vi "Datalog V1.0.vi"(11 "notifiers in":T1) -> ()   [LabVIEW 2022 SP3]
uses:
  Controls/All Notifer.ctl
  Controls/UI Data.ctl
  Controls/Datalog Control.ctl
  Controls/Root path.ctl
  Controls/All Loop Status.ctl
  Sub VI's/Global 1.vi
panel:
  out "error in":errorcluster
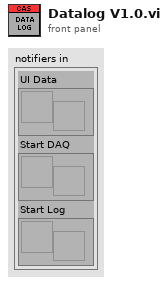
[diagram p1: front panel]
types:
  T1 = typedef "All Notifer.ctl" = cluster{"UI Data":refnum<notifier>, "Start DAQ":refnum<notifier>, "Start Log":refnum<notifier>}
  T2 = typedef "Root path.ctl" = cluster{"Data":path, "Sub VI's":path, "Source code":path}
  T3 = cluster{"in progress?":bool, "DI_ref":refnum<queue>, "Start Log":refnum<notifier>, "tdms ref":refnum<k34>, "AI\nAO\nDO\nTC\nACC\nStrain":refnum<queue>[], "Root Path":T2, "Start time":timestamp}
  T4 = typedef "Datalog Control.ctl" = enum16{"Init", "Poll", "Flush Qs", "Create File", "Log AI", "Log DI", "Log DO", "Log AO", "Close File", "Error", "Exit"}
  T5 = typedef "All Loop Status.ctl" = enum16{"AI", "AO", "DI", "DO", "TC", "Strain", "ACC", "RT", "Log", "Seq", "Sync"}
  T6 = enum16{"Init", "Read 'All'", "Read 'n'", "Read '1'", "Write '1'", "Write 'n'", "Write 'All'"}
  T7 = enum16{"open", "open or create", "create or replace", "create", "open (read-only)"}
  T8 = typedef "All Queue.ctl" = cluster{"AI\nAO\nDO\nTC\nACC\nStrain":refnum<queue>[], "DI":refnum<queue>}
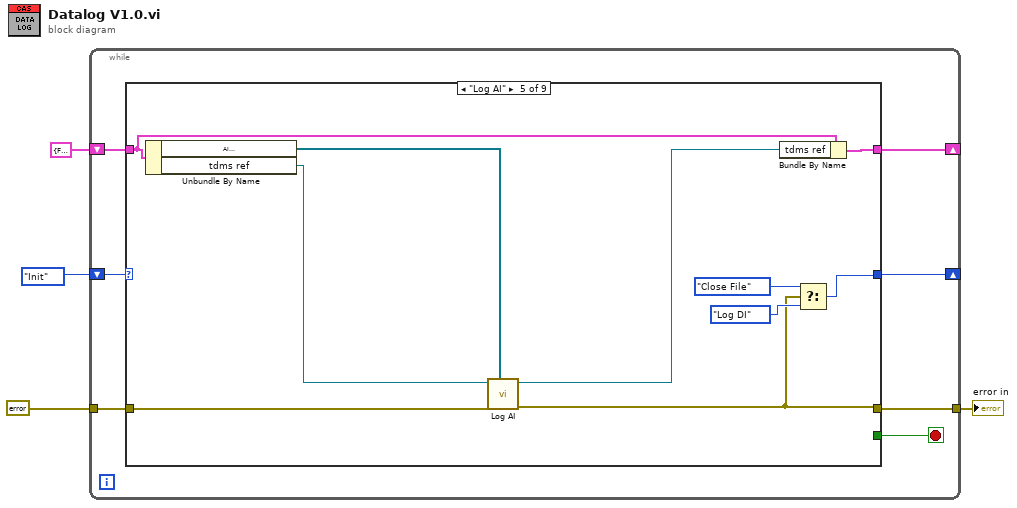
[diagram p0: block diagram]
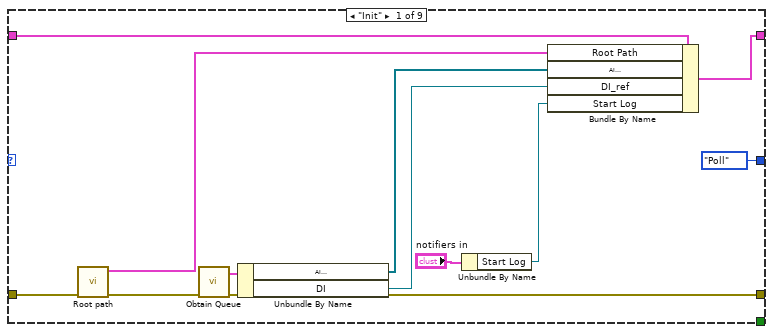
[diagram p2: hidden frame]
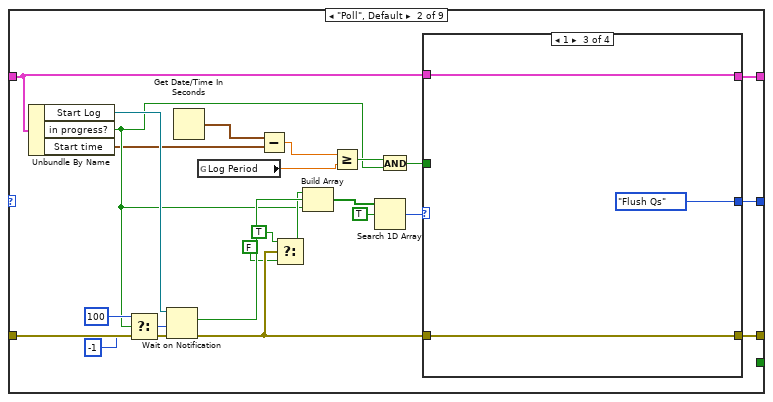
[diagram p3: hidden frame]
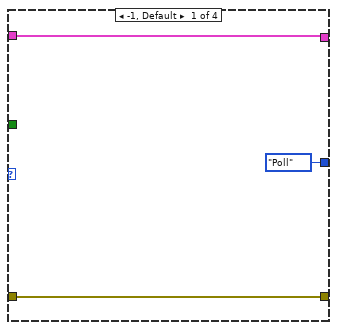
[diagram p4: hidden frame]
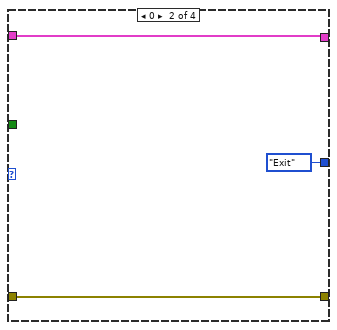
[diagram p5: hidden frame]
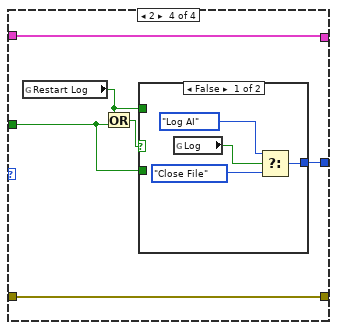
[diagram p6: hidden frame]
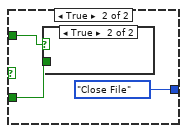
[diagram p7: hidden frame]
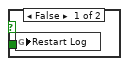
[diagram p8: hidden frame]
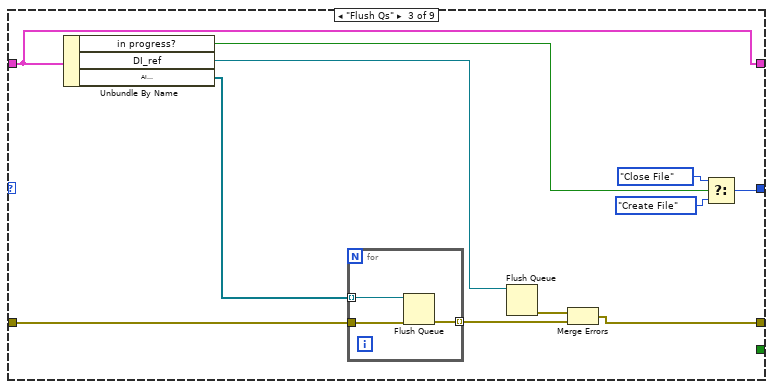
[diagram p9: hidden frame]
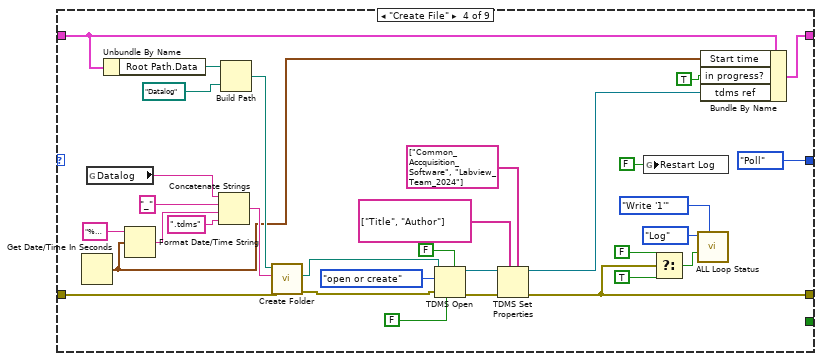
[diagram p10: hidden frame]
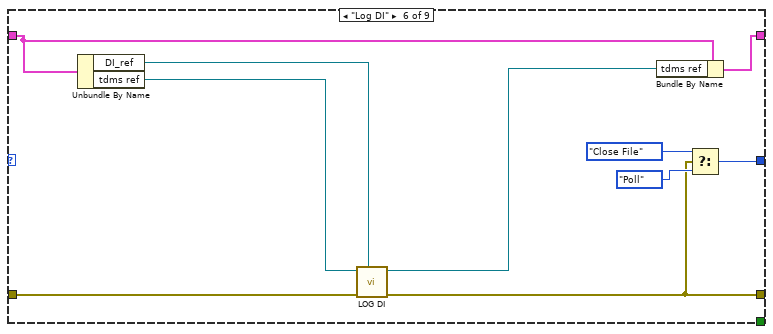
[diagram p11: hidden frame]
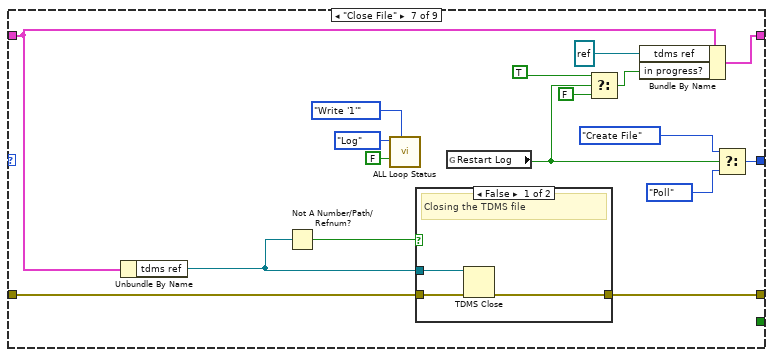
[diagram p12: hidden frame]
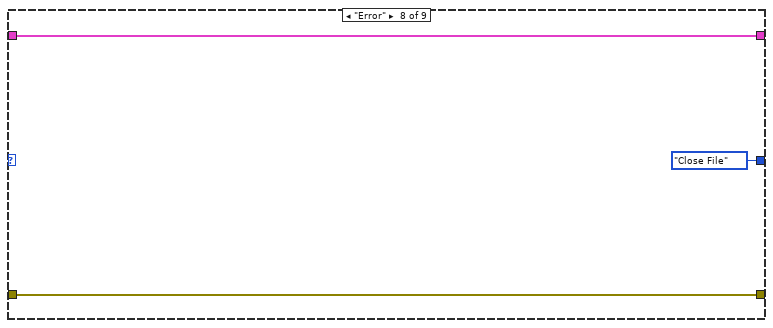
[diagram p14: hidden frame]
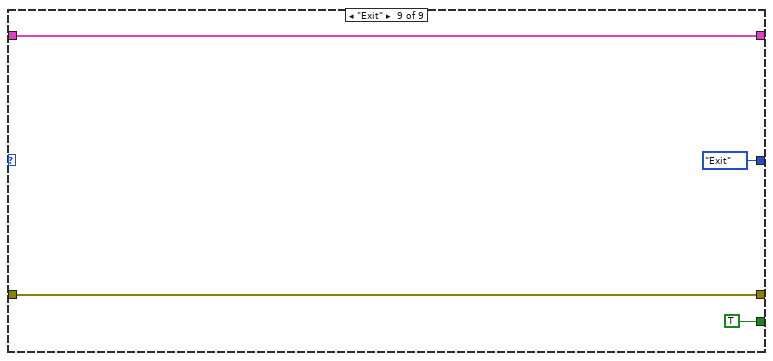
[diagram p15: hidden frame]
diagram:
  n1 = while {
    shift-right: [w10] -> _
    shift-left: Datalog_Control."Init" ("Enum") -> [w11]
    shift-right: [w7] -> _
    shift-left: T3 {"in progress?"=FALSE, "DI_ref"=refnum, "Start Log"=refnum, "tdms ref"=refnum, "AI\nAO\nDO\nTC\nACC\nStrain"=[], "Root Path"={"Data"=path "", "Sub VI's"=path "", "Source code"=path ""}, "Start time"=timestamp(0 s since 1904-01-01)} -> [w8]
    tunnel: errorcluster {"status"=FALSE, "code"=0, "source"=""} ("error in") -> [w6]
    tunnel: [w5] -> w1
    stop <- w9 stop-if-true
    n2 = case shown="\"Log AI\"" w11 {
      tunnel: [Datalog_Control."Poll" ("Enum") w47 w76 Datalog_Control."Poll" ("f") w120 w128 w141 Datalog_Control."Close File" ("f") Datalog_Control."Exit" ("f")] -> w10
      tunnel: [_ _ _ _ _ _ _ _ TRUE] -> w9
      tunnel: w8 -> [w19 w39 w72 w98 w122 w132 w148 w160 w161]
      tunnel: [w20 w40 w72 w106 w123 w133 w149 w160 w161] -> w7
      tunnel: w6 -> [w14 w46 w81 w92 w126 w136 w151 w158 w163]
      tunnel: [w22 w41 w77 w89 w117 w127 w150 w158 w163] -> w5
      frame "Init" {
        n3 = call "Root path.vi"("error in (no error)"=w14) -> ("error out"=w13:errorcluster, "Root Path"=w12:T2)  [unwired: 9 in]
        n4 = call "Obtain Queue.vi"("error in"=w13) -> ("error out"=w22:errorcluster, "Queue ref"=w21:T8)  [unwired: 9 in]
        n5 = Unbundle By Name(w21) -> ("AI\nAO\nDO\nTC\nACC\nStrain"=w15:refnum<queue>[], "DI"=w18:refnum<queue>)
        n6 = Unbundle By Name("notifiers in") -> ("Start Log"=w16:refnum<notifier>)
        n7 = Bundle By Name(cluster=w19, "Root Path"=w12, "AI\nAO\nDO\nTC\nACC\nStrain"=w15, "DI_ref"=w18, "Start Log"=w16) -> (w20:T3)
      }
      frame "Poll", Default {
        n8 = Unbundle By Name(w39) -> ("Start Log"=w42:refnum<notifier>, "in progress?"=w27:bool, "Start time"=w25:timestamp)
        n9 = Select(t=100, s=w27, f=-1 ("timeout in ms (-1)")) -> (s? t:f=w43:i32)
        n10 = Wait on Notification(notifier=w42, timeout in ms (-1)=w43, error in (no error)=w46) -> (notification=w35:bool, error out=w34:errorcluster)  [unwired: 1 in, 2 out]
        n11 = Get Date/Time In Seconds() -> (seconds since 1Jan1904=w26:timestamp)
        n12 = global read "Global 1.vi" "Log Period"() -> (w24:dbl)
        n13 = Subtract(x=w26, y=w25) -> (x-y=w29:dbl)
        n14 = Select(t=TRUE, s=w34, f=FALSE) -> (s? t:f=w31:bool)
        n15 = Build Array(w31, w35, w27) -> (w36:bool[])
        n16 = Greater Or Equal?(x=w29, y=w24) -> (x >= y?=w30:bool)
        n17 = Search 1D Array(1D array=w36, element=TRUE) -> (index of element=w37:i32)  [unwired: 1 in]
        n18 = And(x=w30, y=w27) -> (x .and. y?=w28:bool)
        n19 = case shown="1" w37 {
          tunnel: [Datalog_Control."Poll" ("Enum") Datalog_Control."Exit" ("t") Datalog_Control."Flush Qs" ("Enum") w60] -> w47
          tunnel: w34 -> [w48 w51 w55 w61]
          tunnel: [w48 w51 w55 w61] -> w41
          tunnel: [w50 w52 w54 w62] -> w40
          tunnel: w39 -> [w50 w52 w54 w62]
          tunnel: w28 -> [_ _ _ w58]
          frame -1, Default {
          }
          frame 0 {
          }
          frame 1 {
          }
          frame 2 {
            n20 = global read "Global 1.vi" "Restart Log"() -> (w57:bool)
            n21 = Or(x=w57, y=w58) -> (x .or. y?=w59:bool)
            n22 = case shown="False" w59 {
              tunnel: [w66 Datalog_Control."Close File" ("t")] -> w60
              tunnel: w58 -> [_ w68]
              tunnel: w57 -> [_ w67]
              frame False {
                n23 = global read "Global 1.vi" "Log"() -> (w63:bool)
                n24 = Select(t=Datalog_Control."Log AI" ("Enum"), s=w63, f=Datalog_Control."Close File" ("t")) -> (s? t:f=w66:T4)
              }
              frame True {
                n25 = case shown="True" w67 {
                  tunnel: w68 -> [w70 _]
                  frame False {
                    n26 = global write "Global 1.vi" "Restart Log"(w70) -> ()
                  }
                  frame True {
                  }
                }
              }
            }
          }
        }
      }
      frame "Flush Qs" {
        n27 = Unbundle By Name(w72) -> ("in progress?"=w75:bool, "DI_ref"=w79:refnum<queue>, "AI\nAO\nDO\nTC\nACC\nStrain"=w71:refnum<queue>[])
        n28 = for {
          tunnel: w81 -> [w84]
          tunnel: [w83] -> w80 mode=indexing
          tunnel: w71 -> [w82] mode=indexing
          n29 = Flush Queue(queue=w82, error in (no error)=w84) -> (error out=w83:errorcluster)  [unwired: 2 out]
        }
        n30 = Flush Queue(queue=w79) -> (error out=w78:errorcluster)  [unwired: 1 in, 2 out]
        n31 = Merge Errors(w78, w80) -> (w77:errorcluster)
        n32 = Select(t=Datalog_Control."Close File" ("Enum"), s=w75, f=Datalog_Control."Create File") -> (s? t:f=w76:T4)
      }
      frame "Create File" {
        n33 = Get Date/Time In Seconds() -> (seconds since 1Jan1904=w90:timestamp)
        n34 = global read "Global 1.vi" "Datalog"() -> (w100:string)
        n35 = Unbundle By Name(w98) -> ("Root Path.Data"=w97:path)
        n36 = Format Date/Time String(time format string (%c)="%Y_%b_%d_%Hh_%Mm_%Ssec", seconds (now)=w90) -> (date/time string=w110:string)  [unwired: 1 in]
        n37 = Concatenate Strings(w100, "_" ("string"), w110, ".tdms" ("string")) -> (w94:string)
        n38 = Build Path(base path=w97, name or relative path=path "Datalog" ("base path")) -> (appended path=w95:path)
        n39 = call "Create Folder.vi"("error in (no error)"=w92, "File Name"=w94, "Base Path"=w95) -> ("error out"=w91:errorcluster, "Result File path"=w93:path)  [unwired: 6 in, 1 out]
        n40 = TDMS Open(5:FALSE ("create index file? (T)"), 6:FALSE ("disable buffering? (T)"), 8:w91, 10:T7."open or create" ("operation (0:open)"), 11:w93) -> (0:w115:errorcluster, 3:w116:refnum<k34>)  [unwired: 2 in]
        n41 = TDMS Set Properties(5:string[] ["Common_Accquisition_Software", "Labview_Team_2024"] ("property names"), 7:string[] ["Title", "Author"] ("property names"), 8:w115, 11:w116) -> (0:w89:errorcluster, 3:w104:refnum<k34>)  [unwired: 4 out]
        n42 = global write "Global 1.vi" "Restart Log"(FALSE ("Restart Log")) -> ()
        n43 = Select(t=FALSE ("Restart Log"), s=w89, f=TRUE) -> (s? t:f=w86:bool)
        n44 = call "ALL Loop Status.vi"("Option"=T6."Write '1'", "Status"=w86, "Loop"=All_Loop_Status."Log") -> ()  [unwired: 6 in, 3 out]
        n45 = Bundle By Name(cluster=w98, "Start time"=w90, "in progress?"=TRUE, "tdms ref"=w104) -> (w106:T3)
      }
      frame "Log AI" {
        n46 = Unbundle By Name(w122) -> ("AI\nAO\nDO\nTC\nACC\nStrain"=w125:refnum<queue>[], "tdms ref"=w124:refnum<k34>)
        n47 = call "Log AI.vi"("AI\nAO\nDO\nTC\nACC\nStrain"=w125, "error in"=w126, "tdms file out"=w124) -> ("error out"=w117:errorcluster, "tdms ref out"=w121:refnum<k34>)  [unwired: 7 in]
        n48 = Bundle By Name(cluster=w122, "tdms ref"=w121) -> (w123:T3)
        n49 = Select(t=Datalog_Control."Close File" ("f"), s=w117, f=Datalog_Control."Log DI") -> (s? t:f=w120:T4)
      }
      frame "Log DI" {
        n50 = Unbundle By Name(w132) -> ("DI_ref"=w135:refnum<queue>, "tdms ref"=w134:refnum<k34>)
        n51 = call "LOG DI.vi"("tdms file in"=w134, "error in"=w136, "DI_queue"=w135) -> ("tdms file out"=w131:refnum<k34>, "error out"=w127:errorcluster)  [unwired: 6 in]
        n52 = Bundle By Name(cluster=w132, "tdms ref"=w131) -> (w133:T3)
        n53 = Select(t=Datalog_Control."Close File" ("f"), s=w127, f=Datalog_Control."Poll") -> (s? t:f=w128:T4)
      }
      frame "Close File" {
        n54 = Unbundle By Name(w148) -> ("tdms ref"=w153:refnum<k34>)
        n55 = Not A Number/Path/Refnum?(number/path/refnum=w153) -> (NaN/Path/Refnum?=w152:bool)
        n56 = call "ALL Loop Status.vi"("Option"=T6."Write '1'", "Status"=FALSE, "Loop"=All_Loop_Status."Log") -> ()  [unwired: 6 in, 3 out]
        n57 = case shown="False" w152 {
          tunnel: [w156 w157] -> w150
          tunnel: w153 -> [w155 _]
          tunnel: w151 -> [w154 w157]
          frame False {
            # "Closing the TDMS file"
            n58 = TDMS Close(8:w154, 11:w155) -> (0:w156:errorcluster)  [unwired: 1 out]
          }
          frame True {
          }
        }
        n59 = global read "Global 1.vi" "Restart Log"() -> (w140:bool)
        n60 = Select(t=TRUE ("in progress?"), s=w140, f=FALSE) -> (s? t:f=w137:bool)
        n61 = Bundle By Name(cluster=w148, "tdms ref"=refnum<k34> refnum, "in progress?"=w137) -> (w149:T3)
        n62 = Select(t=Datalog_Control."Create File" ("f"), s=w140, f=Datalog_Control."Poll") -> (s? t:f=w141:T4)
      }
      frame "Error" {
      }
      frame "Exit" {
      }
    }
  }
  "error in" <- w1
